vi "CheckReplyError.vi"(3 "error in":errorcluster, 4 "Response":T1, 5 "Error String":string) -> (0 "error out":errorcluster, 1 "URI":string, 2 "Registered?":bool)   [LabVIEW 2013]
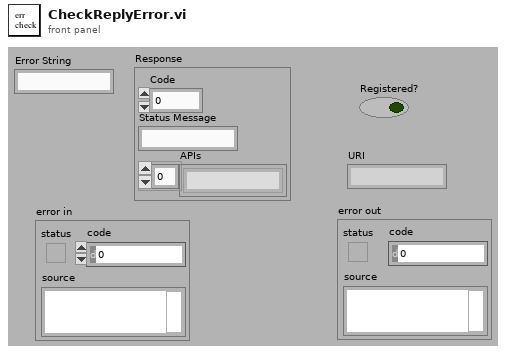
[diagram p1: front panel]
types:
  T1 = cluster{"Code":i32, "Status Message":string, "APIs":string[]}
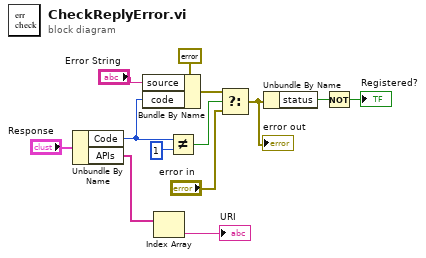
[diagram p0: block diagram]
diagram:
  n1 = Unbundle By Name("Response") -> ("Code"=w4:i32, "APIs"=w8:string[])
  n2 = Bundle By Name(cluster=errorcluster {"status"=TRUE, "code"=0, "source"=""} ("error out"), "source"="Error String", "code"=w4) -> (w5:errorcluster)
  n3 = Index Array(array=w8) -> (element=→"URI":string)  [unwired: 1 in]
  n4 = Not Equal?(x=w4, y=1) -> (x != y?=w3:bool)
  n5 = Select(t=w5, s=w3, f="error in") -> (s? t:f=w11:errorcluster)
  "error out" <- w11
  n6 = Unbundle By Name(w11) -> ("status"=w12:bool)
  n7 = Not(x=w12) -> (.not. x?=→"Registered?":bool)
